vi "Configure ECAT Generic Slave Wrapper.vi"(8 "error in":errorcluster, 10 "Distributed Clock":bool, 11 "IOV ref":refnum<k21>) -> (0 "error out":errorcluster, 2 "Distributed Clock out":bool, 3 "IOV ref out":refnum<k21>)   [LabVIEW 2019, in "SEECD Engine.lvlib"]
uses:
  SEECD Engine.lvlib
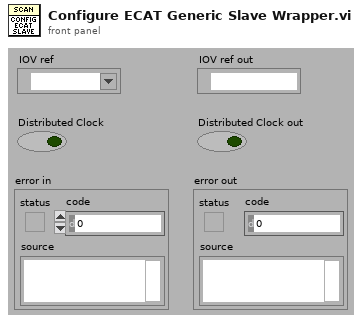
[diagram p1: front panel]
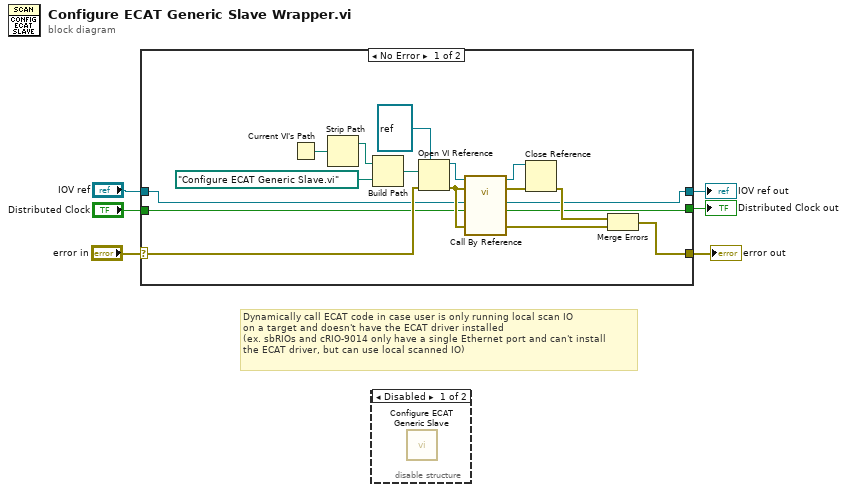
[diagram p0: block diagram]
diagram:
  # "Dynamically call ECAT code in case user is only running local scan IO\non a target and doesn't have the ECAT driver installed\n(ex. sbRIOs and cRIO-9014 only have a single Ethernet port and can't install\nthe ECAT driver, but can use local scanned IO)"
  n1 = case shown="No Error" "error in" {
    selector: "error in" -> [w11 w26]
    tunnel: [w12 w26] -> w6
    tunnel: [w10 w25] -> w4
    tunnel: [w9 w24] -> w3
    tunnel: "IOV ref" -> [w8 w25]
    tunnel: "Distributed Clock" -> [w7 w24]
    frame No Error {
      n2 = Current VI's Path() -> (path=w14:path)
      n3 = Strip Path(path=w14) -> (stripped path=w16:path)  [unwired: 1 out]
      n4 = Build Path(base path=w16, name or relative path=path "Configure ECAT Generic Slave.vi" ("vi path")) -> (appended path=w17:path)
      n5 = Open VI Reference(type specifier VI Refnum (for type only)=refnum<vi> refnum, vi path=w17, error in (no error)=w11) -> (vi reference=w19:refnum<vi>, error out=w18:errorcluster)  [unwired: 3 in]
      n6 = call-by-ref "?"(reference=w19, error in=w18, "error in"=w18, "Distributed Clock"=w7, "IOV ref"=w8) -> (reference out=w21:refnum<vi>, error out=w20:errorcluster, 0:"error out"=w22:errorcluster, "Distributed Clock out"=w9:bool, "IOV ref out"=w10:refnum<k21>)  [unwired: 6 in]
      n7 = Close Reference(reference=w21, error in (no error)=w20) -> (error out=w23:errorcluster)
      n8 = Merge Errors(w23, w22) -> (w12:errorcluster)
    }
    frame Error {
    }
  }
  "error out" <- w6
  "IOV ref out" <- w4
  "Distributed Clock out" <- w3
  n9 = disable-structure shown="Disabled" {
    frame Disabled {
      n10 = call "Configure ECAT Generic Slave.vi"() -> ()  [unwired: 9 in, 3 out]
    }
    frame Enabled {
    }
  }
